vi "GeneralModbus.vi"(9 "VISA resource name":refnum<visa-resource-name>) -> (1 "error out":errorcluster, 2 "TemperatureValue":string)   [LabVIEW 2017]
uses:
  <vilib>/NI/Modbus Library/API/Wrapper/Create Serial Master.vi
  <vilib>/NI/Modbus Library/API/Master/Modbus Master.lvclass
  <vilib>/NI/Modbus Library/API/Wrapper/API Main.lvlib
panel:
  out "HumidityValue":string
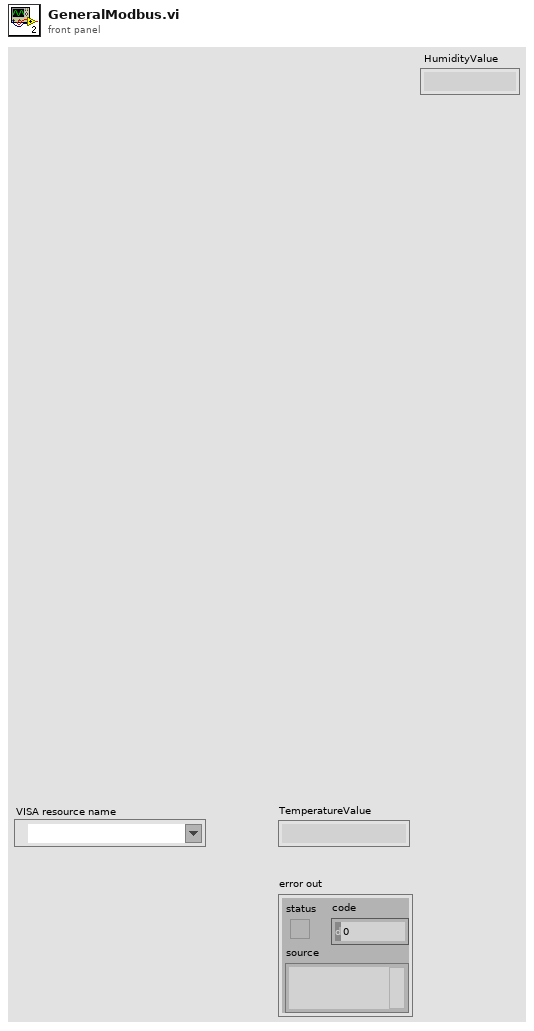
[diagram p1: front panel]
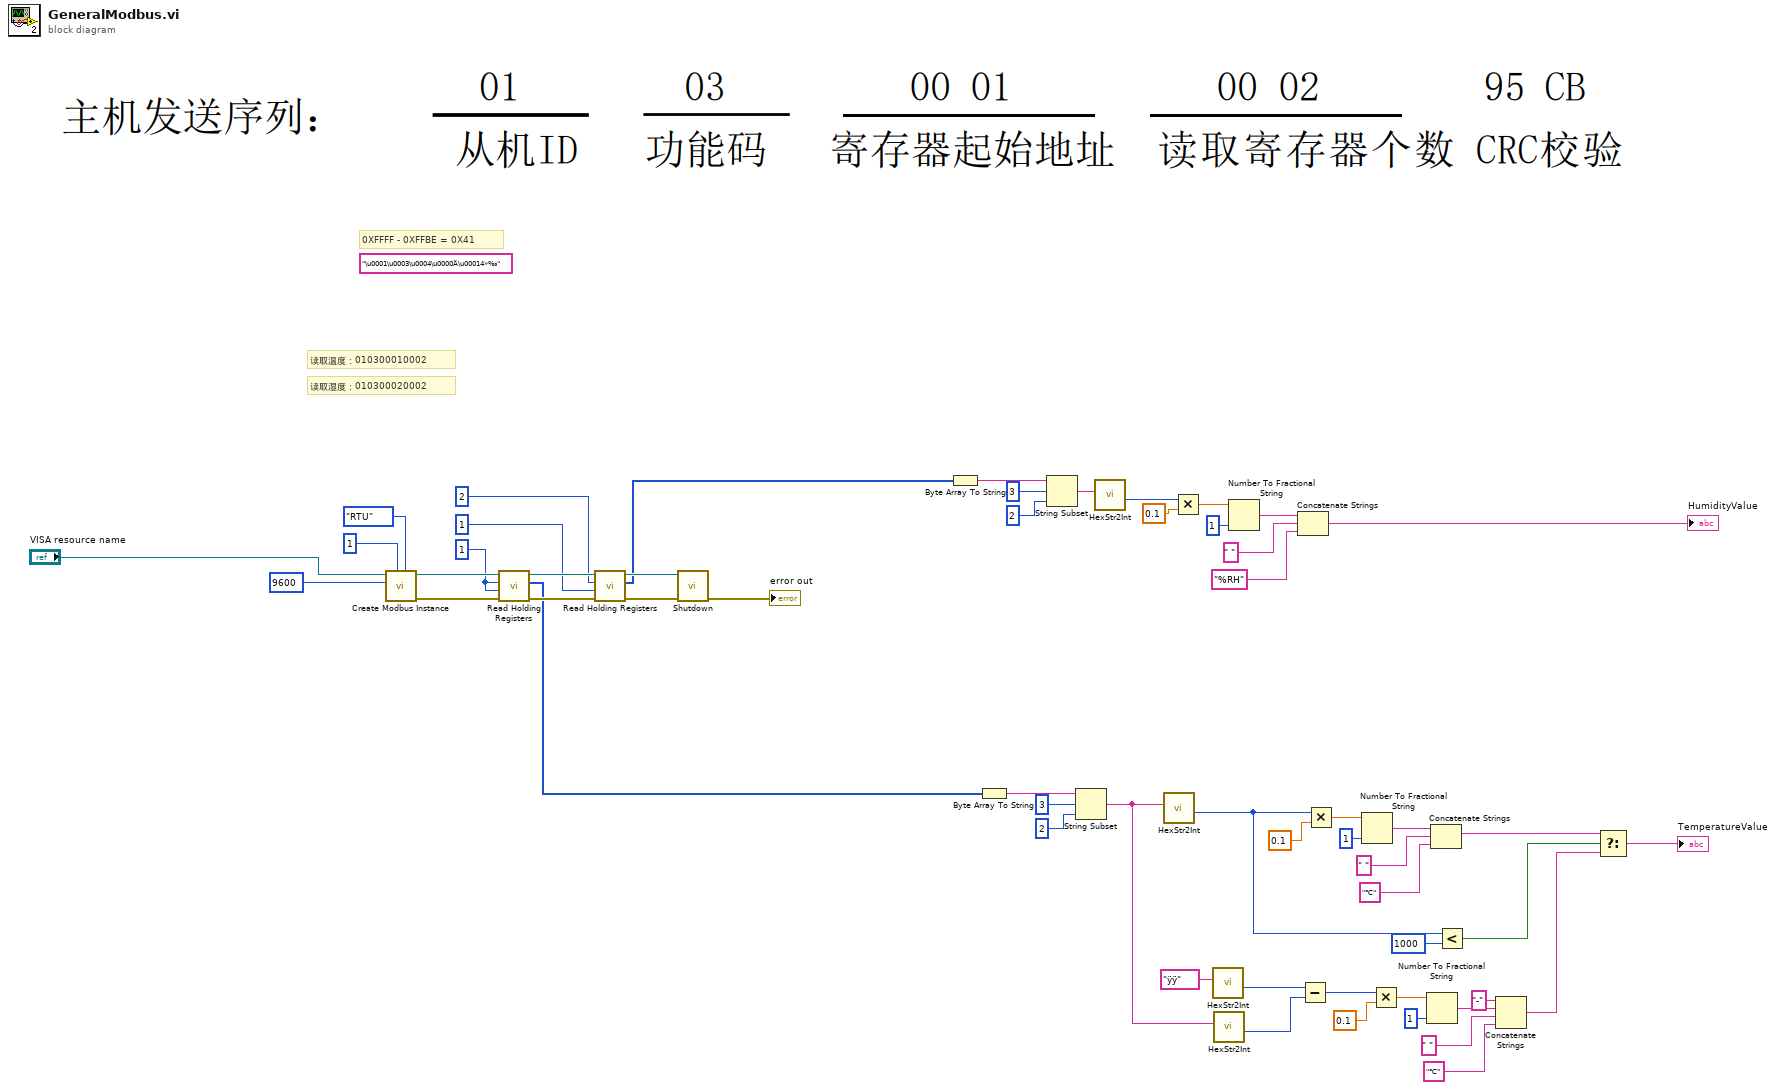
[diagram p0: block diagram]
diagram:
  w29 = u16 1 ("starting address")
  (unwired) "\u0001\u0003\u0004\u0000Ä\u00014»‰"
  # "0XFFFF - 0XFFBE = 0X41"
  # "读取湿度：010300020002"
  # "读取温度：010300010002"
  n1 = call-poly <vilib>:"Create Modbus Instance.vi"("serial type"=enum16{"RTU", "ASCII"}."RTU", "unit ID"=u8 1, "baud rate"=u32 9600, "VISA resource name"="VISA resource name") -> ("error out"=w30:errorcluster, "serial master instance"=w31:refnum<class "Modbus Master.lvclass">)  [unwired: 6 in]
  n2 = call-dynamic "Read Holding Registers.vi"("error in"=w30, "number of inputs"=w29, "starting address"=w29, "Modbus master in"=w31) -> ("error out"=w27:errorcluster, "register values"=w22:u16[], "Modbus master out"=w28:refnum<class "Modbus Master.lvclass">)  [unwired: 5 in]
  n3 = call-dynamic "Read Holding Registers.vi"("error in"=w27, "number of inputs"=u16 1 ("starting address"), "starting address"=u16 2, "Modbus master in"=w28) -> ("error out"=w25:errorcluster, "register values"=w2:u16[], "Modbus master out"=w26:refnum<class "Modbus Master.lvclass">)  [unwired: 5 in]
  n4 = call-dynamic "Shutdown.vi"("error in"=w25, "Modbus master in"=w26) -> ("error out"=→"error out":errorcluster)  [unwired: 9 in]
  n5 = Byte Array To String(unsigned byte array=w2) -> (string=w11:string)
  n6 = Byte Array To String(unsigned byte array=w22) -> (string=w21:string)
  n7 = String Subset(string=w11, offset (0)=3 ("偏移量(0)"), length (rest)=2 ("长度（剩余）")) -> (substring=w13:string)
  n8 = String Subset(string=w21, offset (0)=3 ("偏移量(0)"), length (rest)=2 ("长度（剩余）")) -> (substring=w14:string)
  n9 = call "HexStr2Int.vi"("十六进制字符串"=w13) -> ("数字"=w12:u32)  [unwired: 10 in]
  n10 = call "HexStr2Int.vi"("十六进制字符串"=w14) -> ("数字"=w16:u32)  [unwired: 10 in]
  n11 = Multiply(x=w12, y=0.1) -> (x*y=w6:dbl)
  n12 = call "HexStr2Int.vi"("十六进制字符串"="ÿÿ") -> ("数字"=w46:u32)  [unwired: 10 in]
  n13 = call "HexStr2Int.vi"("十六进制字符串"=w14) -> ("数字"=w45:u32)  [unwired: 10 in]
  n14 = Number To Fractional String(number=w6, precision (6)=i16 1 ("精度(6)")) -> (F-format string=w10:string)  [unwired: 2 in]
  n15 = Concatenate Strings(w10, " " ("字符串"), "%RH" ("字符串")) -> (→"HumidityValue":string)
  n16 = Subtract(x=w46, y=w45) -> (x-y=w38:u32)
  n17 = Multiply(x=w16, y=0.1) -> (x*y=w52:dbl)
  n18 = Number To Fractional String(number=w52, precision (6)=i16 1 ("精度(6)")) -> (F-format string=w48:string)  [unwired: 2 in]
  n19 = Multiply(x=w38, y=0.1) -> (x*y=w40:dbl)
  n20 = Number To Fractional String(number=w40, precision (6)=i16 1 ("精度(6)")) -> (F-format string=w44:string)  [unwired: 2 in]
  n21 = Concatenate Strings(w48, " " ("字符串"), "℃" ("字符串")) -> (w18:string)
  n22 = Less?(x=w16, y=u32 1000) -> (x < y?=w19:bool)
  n23 = Concatenate Strings("-" ("字符串"), w44, " " ("字符串"), "℃" ("字符串")) -> (w17:string)
  n24 = Select(t=w18, s=w19, f=w17) -> (s? t:f=→"TemperatureValue":string)
